vi "Close.vi"(8 "error in":errorcluster, 11 "FileHandler in":refnum<class "FileHandler.lvclass">) -> (0 "error out":errorcluster, 3 "FileHandler out":refnum<class "FileHandler.lvclass">)   [LabVIEW 2020, in "hse-logger.lvlib" / "FileHandler.lvclass"]
doc: "Closes the log-file. This method should be called when the ``Logger`` gets closed or the handler is removed from the ``Logger``.\n\n____\nHAMPEL SOFTWARE ENGINEERING v2.0.6 (2021-04-15 11:38)"
uses:
  FileHandler.lvclass
  FileHandler.lvclass/FileHandler.ctl
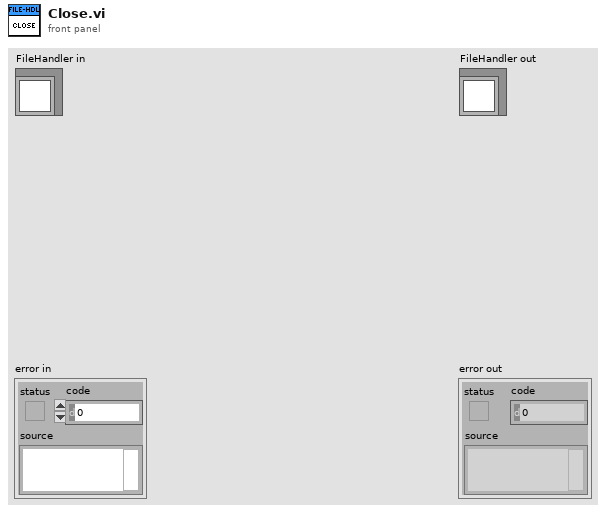
[diagram p1: front panel]
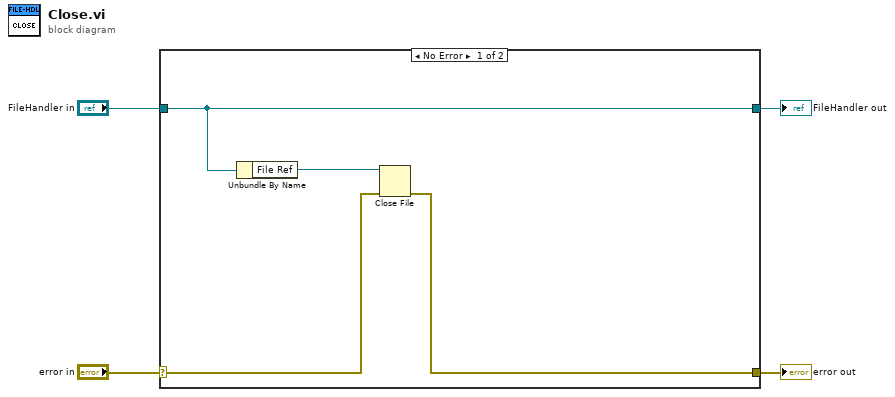
[diagram p0: block diagram]
diagram:
  n1 = case shown="No Error" "error in" {
    selector: "error in" -> [w6 w10]
    tunnel: [w5 w10] -> w3
    tunnel: [w8 w9] -> w1
    tunnel: "FileHandler in" -> [w8 w9]
    frame No Error {
      n2 = Unbundle By Name(w8) -> ("File Ref"=w7:refnum<file>)
      n3 = Close File(refnum=w7, error in=w6) -> (error out=w5:errorcluster)  [unwired: 1 out]
    }
    frame Error {
    }
  }
  "error out" <- w3
  "FileHandler out" <- w1
